vi "test for a regexp list.vi"(6 "quote specials":bool, 10 "string":string="aaa bbb.ccc", 11 "regexps":string[](array[string])=["aaa", "bbb", "aaa bbb.ccc", "aaa bbb ccc", "dddd"]) -> (0 "whole match":string, 1 "match found":bool, 2 "matching string index":i32, 3 "matching regexp":string)   [LabVIEW 2015]
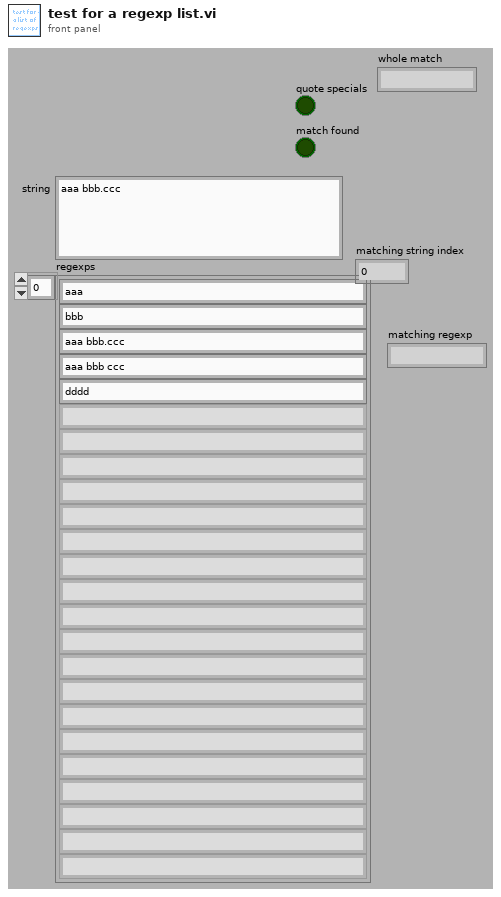
[diagram p1: front panel]
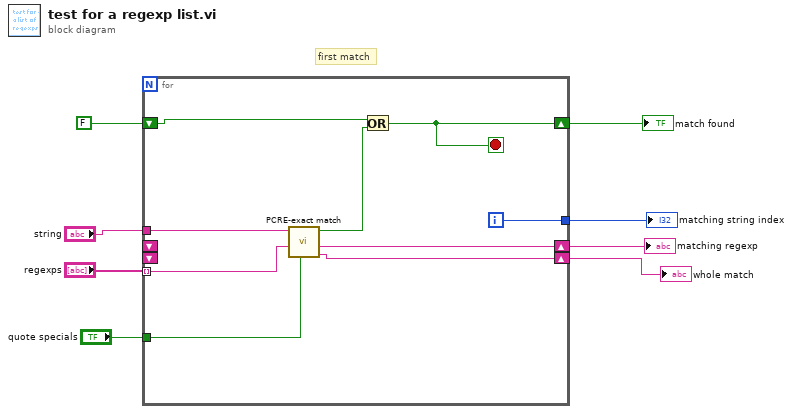
[diagram p0: block diagram]
diagram:
  # "first match"
  n1 = for {
    tunnel: "regexps" -> [w10] mode=indexing
    tunnel: "string" -> [w11]
    shift-right: [w10] -> w6
    shift-left: _ -> [_]
    shift-right: [w15] -> w5
    shift-left: FALSE -> [w14]
    tunnel: [w13] -> w3
    tunnel: "quote specials" -> [w12]
    shift-right: [w9] -> w1
    shift-left: _ -> [_]
    i -> [w13]
    stop <- w15 stop-if-true
    n2 = call "PCRE-exact match.vi"("quote specials"=w12, "regular expression"=w10, "input string"=w11) -> ("whole match"=w9:string, "exact match"=w16:bool)  [unwired: 6 in, 1 out]
    n3 = Or(x=w14, y=w16) -> (x .or. y?=w15:bool)
  }
  "matching regexp" <- w6
  "match found" <- w5
  "matching string index" <- w3
  "whole match" <- w1
